vi "Event Handler.vi"(0 "uService Template in":refnum<class "Run Config Manager.lvclass">, 5 "Event type":T1=enum."Message", 7 "Item Name":string, 9 "Data":variant, 11 "error in (no error)":errorcluster) -> (4 "uService Template out":refnum<class "Run Config Manager.lvclass">, 15 "error out":errorcluster)   [LabVIEW 2026, in "TALOS.lvlib" / "Run Config Manager.lvlib" / "Run Config Manager.lvclass"]
uses:
  Run Config Manager.lvclass
  C:/LabVIEW Code/TALOS/talos/Father of all uServices/Father of all uServices/Father of all uServices.lvclass
  C:/LabVIEW Code/TALOS/builds/Actor Framework PPL/Actor Framework.lvlibp/1abvi3w/vi.lib/ActorFramework/Actor/Actor.lvclass
  Father of all uServices/Father of all uServices/Event Handler Items.ctl
  Ancestor/Ancestor/Ancestor.lvclass/Ancestor.ctl
  Guardian/Guardian/Buttons_UI.ctl
  Guardian/Guardian Messages/Button Pressed Msg/Button Pressed Msg.lvclass/Button Pressed Msg.ctl
  FGV/Error Memory/Get Error Description.vi
  Support VIs/Get PC name.vi
  Ancestor/Ancestor/Read ID.vi
  Support VIs/Get Class Name.vi
  <vilib>/Utility/error.llb/Clear Errors.vi
  FGV/Error Memory/Error Memory Core.vi
  <vilib>/AdvancedString/Delimited String to 1D String Array.vi
  <vilib>/AdvancedString/Delimited String to 1D String Array (string).vi
  Support VIs/Circus Root Path.vi
  FGV/Error Memory/Error Crt Lvl checker.vi
  FGV/Error Memory/Error Memory Core.vi/40c8088d-b597-4017-91af-faa98e00292e.vi
  FGV/Error Memory/Error Memory Core.vi/d4a3ab98-063c-4e44-b43d-fbdcfe6c2be2.vi
  Support VIs/Global Memory.vi
  <vilib>/Utility/LVClass/Get LV Class Name.vi
  Support VIs/Is in Packed Library.vi
  Support VIs/TALOS Root path.vi
  Support VIs/Read CSV worksheet.vi
  Support VIs/Global Constants.vi
  <vilib>/Utility/error.llb/General Error Handler.vi
  builds/Actor Framework PPL/Actor Framework.lvlibp/1abvi3w/vi.lib/ActorFramework/Message Enqueuer/Enqueue.vi
  Ancestor/Ancestor/Ancestor.lvclass
  <vilib>/Comparison/Equal/Equal Functor/Equal Functor.lvclass
  Guardian/Guardian Messages/Button Pressed Msg/Button Pressed Msg.lvclass
  Father of all uServices/Father of all uServices/Father of all uServices.lvclass
  TALOS.lvlib
  Guardian/Guardian/Guardian.lvclass
  builds/Actor Framework PPL/Actor Framework.lvlibp/1abvi3w/vi.lib/ActorFramework/Actor/Actor.lvclass
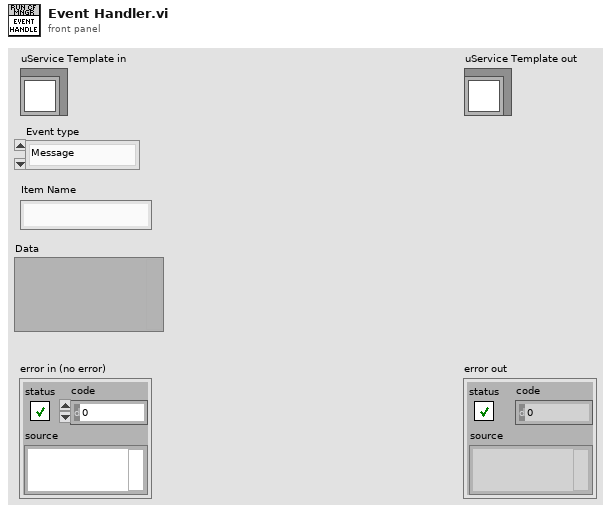
[diagram p1: front panel]
types:
  T1 = typedef "TALOS.lvlib/Father of all uServices.lvlib/Father of all uServices.lvclass/Event Handler Items.ctl" = enum16{"Button Pressed", "Message", "Ready to launch?", "Safe Mode", "Start RUN", "Stop RUN"}
  T2 = typedef "TALOS.lvlib/Guardian.lvlib/Guardian.lvclass/Buttons_UI.ctl" = enum16{"Start uService", "Kill uService", "Stop uService", "Stop", "Start online checks", "Stop online checks", "Send Pat to all GDs", "Reload INI files", "Update from GIT", "RUN", "Reset ABORT", "Check Bearer", "Send I Exist", "Change Run Config", "Add uSs from Config", "Realign uSs from Config", "Send Run Config to GD"}
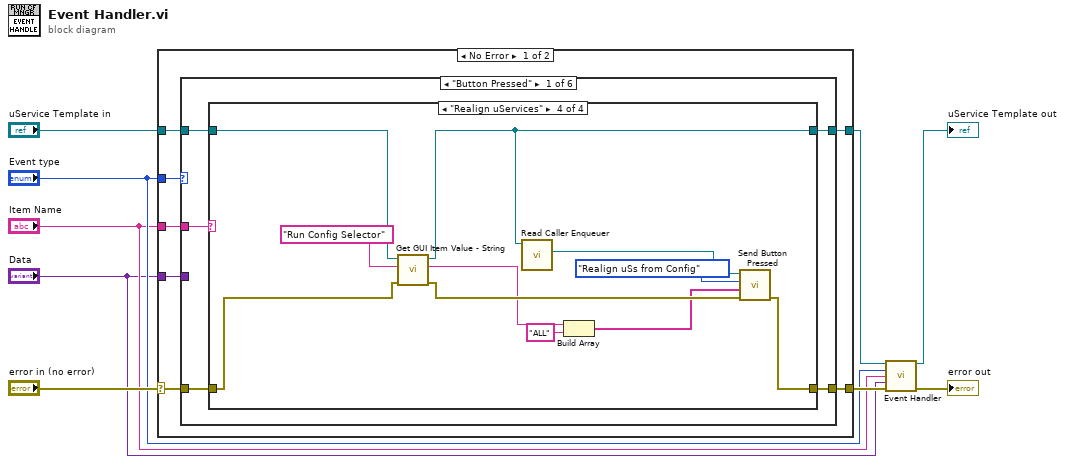
[diagram p0: block diagram]
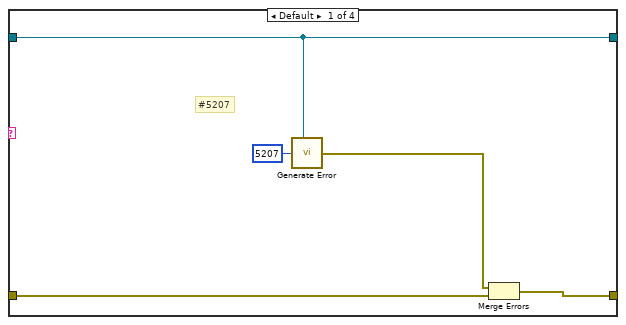
[diagram p2: hidden frame]
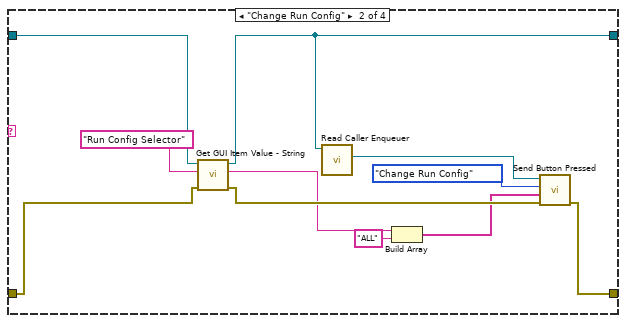
[diagram p3: hidden frame]
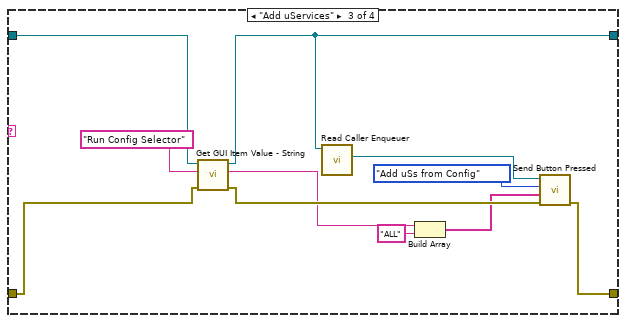
[diagram p4: hidden frame]
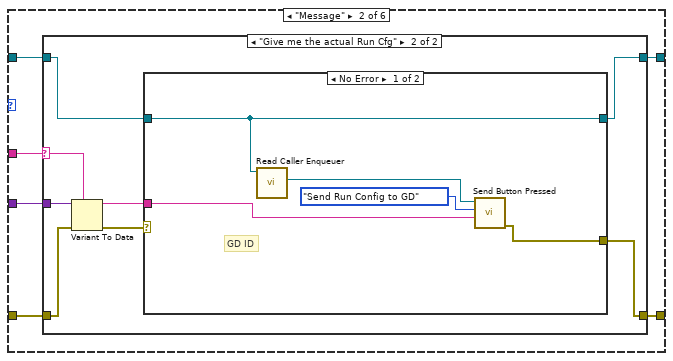
[diagram p5: hidden frame]
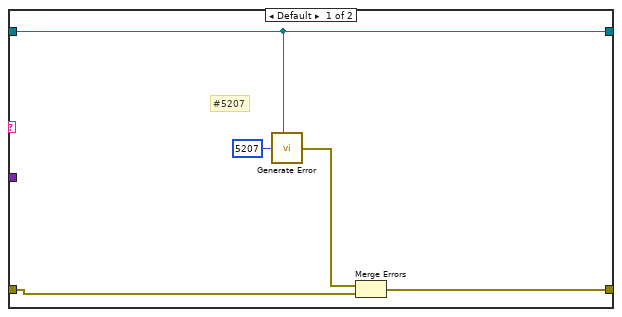
[diagram p6: hidden frame]
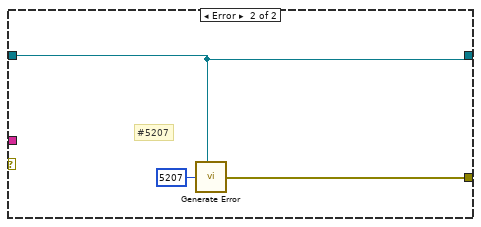
[diagram p7: hidden frame]
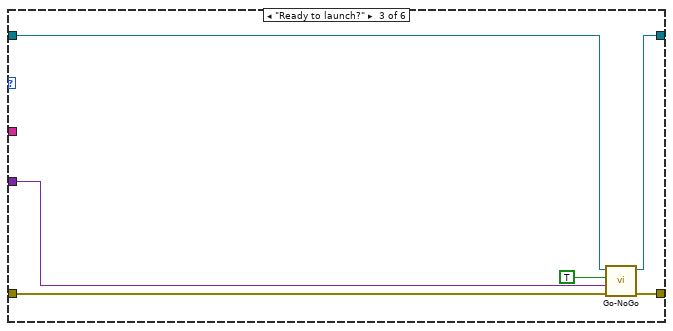
[diagram p8: hidden frame]
diagram:
  n1 = case shown="No Error" "error in (no error)" {
    selector: "error in (no error)" -> [w13 w100]
    tunnel: [w12 w100] -> w7
    tunnel: "uService Template in" -> [w15 w99]
    tunnel: [w14 w99] -> w4
    tunnel: "Event type" -> [w16 _]
    tunnel: "Item Name" -> [w11 _]
    tunnel: "Data" -> [w10 _]
    frame No Error {
      n2 = case shown="\"Button Pressed\"" w16 {
        tunnel: w15 -> [w21 w65 w89 w94 w96 w98]
        tunnel: [w20 w61 w92 w94 w96 w98] -> w14
        tunnel: w13 -> [w17 w62 w90 w93 w95 w97]
        tunnel: [w18 w60 w91 w93 w95 w97] -> w12
        tunnel: w11 -> [w19 w64 _ _ _ _]
        tunnel: w10 -> [_ w63 w87 _ _ _]
        frame "Button Pressed" {
          n3 = case shown="\"Realign uServices\"" w19 {
            tunnel: w21 -> [w22 w32 w43 w54]
            tunnel: [w22 w31 w42 w53] -> w20
            tunnel: [w25 w29 w40 w51] -> w18
            tunnel: w17 -> [w26 w30 w41 w52]
            frame Default {
              # "#5207"
              n4 = call "Generate Error.vi"("Class"=w22, "Error Code"=5207) -> ("error out"=w24:errorcluster)  [unwired: 5 in]
              n5 = Merge Errors(w24, w26) -> (w25:errorcluster)
            }
            frame "Change Run Config" {
              n6 = call "Get GUI Item Value - String.vi"("error in (no error)"=w30, "FP Item Name"="Run Config Selector", "uService Template in"=w32) -> ("error out"=w34:errorcluster, "Value"=w33:string, "uService Template out"=w31:refnum<class "Run Config Manager.lvclass">)  [unwired: 6 in]
              n7 = call "Read Caller Enqueuer.vi"("Actor"=w31) -> ("Caller Enqueuer"=w36:refnum<class "Message Enqueuer.lvclass">)  [unwired: 10 in]
              n8 = Build Array(w33, "ALL" ("element")) -> (w28:string[])
              n9 = call "Send Button Pressed.vi"("error in (no error)"=w34, "Data"=w28, "Button"=Buttons_UI."Change Run Config", "Message Enqueuer"=w36) -> ("error out"=w29:errorcluster)  [unwired: 6 in, 1 out]
            }
            frame "Add uServices" {
              n10 = call "Get GUI Item Value - String.vi"("error in (no error)"=w41, "FP Item Name"="Run Config Selector", "uService Template in"=w43) -> ("error out"=w45:errorcluster, "Value"=w44:string, "uService Template out"=w42:refnum<class "Run Config Manager.lvclass">)  [unwired: 6 in]
              n11 = call "Read Caller Enqueuer.vi"("Actor"=w42) -> ("Caller Enqueuer"=w47:refnum<class "Message Enqueuer.lvclass">)  [unwired: 10 in]
              n12 = Build Array(w44, "ALL" ("element")) -> (w39:string[])
              n13 = call "Send Button Pressed.vi"("error in (no error)"=w45, "Data"=w39, "Button"=Buttons_UI."Add uSs from Config", "Message Enqueuer"=w47) -> ("error out"=w40:errorcluster)  [unwired: 6 in, 1 out]
            }
            frame "Realign uServices" {
              n14 = call "Get GUI Item Value - String.vi"("error in (no error)"=w52, "FP Item Name"="Run Config Selector", "uService Template in"=w54) -> ("error out"=w56:errorcluster, "Value"=w55:string, "uService Template out"=w53:refnum<class "Run Config Manager.lvclass">)  [unwired: 6 in]
              n15 = call "Read Caller Enqueuer.vi"("Actor"=w53) -> ("Caller Enqueuer"=w58:refnum<class "Message Enqueuer.lvclass">)  [unwired: 10 in]
              n16 = Build Array(w55, "ALL" ("element")) -> (w50:string[])
              n17 = call "Send Button Pressed.vi"("error in (no error)"=w56, "Data"=w50, "Button"=Buttons_UI."Realign uSs from Config", "Message Enqueuer"=w58) -> ("error out"=w51:errorcluster)  [unwired: 6 in, 1 out]
            }
          }
        }
        frame "Message" {
          n18 = case shown="\"Give me the actual Run Cfg\"" w64 {
            selector: w64 -> [_ w77]
            tunnel: w65 -> [w68 w73]
            tunnel: w63 -> [_ w78]
            tunnel: w62 -> [w66 w76]
            tunnel: [w68 w72] -> w61
            tunnel: [w67 w71] -> w60
            frame Default {
              # "#5207"
              n19 = call "Generate Error.vi"("Class"=w68, "Error Code"=5207) -> ("error out"=w69:errorcluster)  [unwired: 5 in]
              n20 = Merge Errors(w69, w66) -> (w67:errorcluster)
            }
            frame "Give me the actual Run Cfg" {
              n21 = Variant To Data(error in=w76, type=w77, Variant=w78) -> (data=w74:string, error out=w75:errorcluster)
              n22 = case shown="No Error" w75 {
                tunnel: w74 -> [w81 _]
                tunnel: w73 -> [w82 w85]
                tunnel: [w82 w85] -> w72
                tunnel: [w80 w84] -> w71
                frame No Error {
                  # "GD ID"
                  n23 = call "Read Caller Enqueuer.vi"("Actor"=w82) -> ("Caller Enqueuer"=w83:refnum<class "Message Enqueuer.lvclass">)  [unwired: 10 in]
                  n24 = call "Send Button Pressed.vi"("Data"=w81, "Button"=Buttons_UI."Send Run Config to GD", "Message Enqueuer"=w83) -> ("error out"=w80:errorcluster)  [unwired: 7 in, 1 out]
                }
                frame Error {
                  # "#5207"
                  n25 = call "Generate Error.vi"("Class"=w85, "Error Code"=5207) -> ("error out"=w84:errorcluster)  [unwired: 5 in]
                }
              }
            }
          }
        }
        frame "Ready to launch?" {
          n26 = call-dynamic "Go-NoGo.vi"("error in (no error)"=w90, "Go-NoGo Data"=w87, "Go?"=TRUE, "Father of all uServices in"=w89) -> ("error out"=w91:errorcluster, "Father of all uServices out"=w92:refnum<class "Run Config Manager.lvclass">)  [unwired: 6 in]
        }
        frame "Safe Mode" {
        }
        frame "Start RUN" {
        }
        frame "Stop RUN" {
        }
      }
    }
    frame Error {
    }
  }
  n27 = call-parent "Event Handler.vi"("uService Template in"=w4, "Event type"="Event type", "Item Name"="Item Name", "Data"="Data", "error in (no error)"=w7) -> ("uService Template out"=→"uService Template out":refnum<class "Run Config Manager.lvclass">, "error out"=→"error out":errorcluster)  [unwired: 9 in]
